vi "Get Array of Limit Status.vi"(8 "error in (no error)":errorcluster, 11 "Motions in":refnum<class "Motions.lvclass">) -> (0 "error out":errorcluster, 1 "Array of Limit Status cluster":cluster{"Limit -":bool, "Limit +":bool}[](array[cluster]), 2 "Array of Limit Status":bool[](array[boolean]), 3 "Motions out":refnum<class "Motions.lvclass">)   [LabVIEW 2016, in "Hardware.lvlib" / "Motions.lvlib" / "Motions.lvclass"]
uses:
  <userlib>/Common Components/Hardware/Abstract System/Motions/Motions/Motions.lvclass
  <userlib>/Common Components/Hardware/Abstract System/Motions/Motions/Motions.lvclass/Motions.ctl
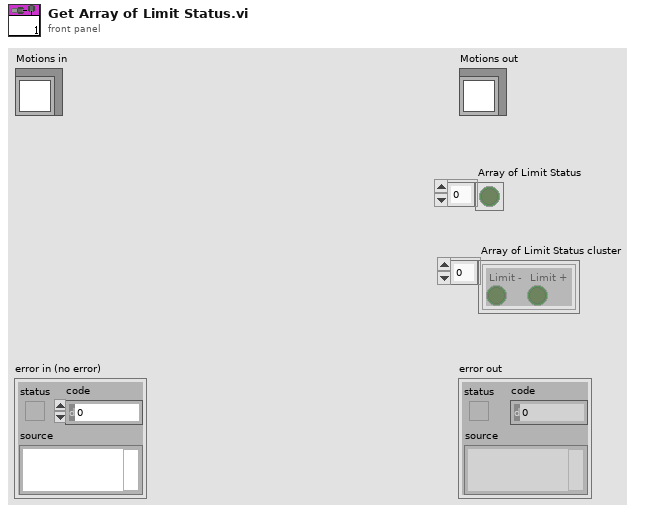
[diagram p1: front panel]
types:
  T1 = cluster{"Connected":bool, "Enabled":bool, "Moving Status":bool, "Soft Moving Status":bool, "Current Pos":dbl, "Target Pos":dbl, "Moving Dir (-1, 0, 1)":i32, "Error Status":bool, "Hard Limit+":bool, "Hard Limit-":bool, "Soft Limit+":bool, "Soft Limit-":bool}[]
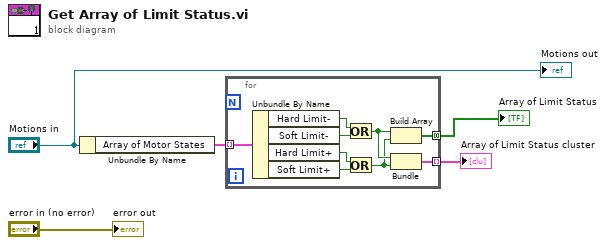
[diagram p0: block diagram]
diagram:
  n1 = Unbundle By Name("Motions in") -> ("Array of Motor States"=w3:T1)
  n2 = for {
    tunnel: w3 -> [w14] mode=indexing
    tunnel: [w9] -> w2 mode=concatenating
    tunnel: [w6] -> w1 mode=indexing
    n3 = Unbundle By Name(w14) -> ("Hard Limit-"=w13:bool, "Soft Limit-"=w12:bool, "Hard Limit+"=w11:bool, "Soft Limit+"=w10:bool)
    n4 = Or(x=w13, y=w12) -> (x .or. y?=w8:bool)
    n5 = Or(x=w11, y=w10) -> (x .or. y?=w7:bool)
    n6 = Build Array(w8, w7) -> (w9:bool[])
    n7 = Bundle(w8, w7) -> (w6:cluster{bool, bool})  [unwired: 1 in]
  }
  "Array of Limit Status" <- w2
  "Array of Limit Status cluster" <- w1
  "error out" <- "error in (no error)"
  "Motions out" <- "Motions in"
